vi "ROS_Read_Motors.vi"(7 "wl_in":T1={"topic port"=0, "Node"="", "topic"="", "type"="", "node port"=0, "error "={"status"=FALSE, "code"=0, "source"=""}, "Direction"=enum."Node", "Update (ms)"=1, "FIFO size"=1}, 8 "error in (no error)":errorcluster, 11 "wr_in":T1={"topic port"=0, "Node"="", "topic"="", "type"="", "node port"=0, "error "={"status"=FALSE, "code"=0, "source"=""}, "Direction"=enum."Node", "Update (ms)"=1, "FIFO size"=1}) -> (0 "error out":errorcluster, 1 "wr":sgl, 2 "wl":sgl, 3 "wr_out":T1={"topic port"=0, "Node"="", "topic"="", "type"="", "node port"=0, "error "={"status"=FALSE, "code"=0, "source"=""}, "Direction"=enum."Node", "Update (ms)"=1, "FIFO size"=1}, 5 "wl_out":T1={"topic port"=0, "Node"="", "topic"="", "type"="", "node port"=0, "error "={"status"=FALSE, "code"=0, "source"=""}, "Direction"=enum."Node", "Update (ms)"=1, "FIFO size"=1})   [LabVIEW 2017]
doc: "Read motors' left and right rotational velocity from ROS topics"
uses:
  <vilib>/Tufts CEEO ROS for LabVIEW Software/ROS/Code/SubVIs/_ROSControl.ctl
  <vilib>/Tufts CEEO ROS for LabVIEW Software/ROS/Code/SubVIs/_ROSDirection.ctl
  <vilib>/Tufts CEEO ROS for LabVIEW Software/ROS/MessageParsing/std_msgs/subs/parse_float32_scalar.vi
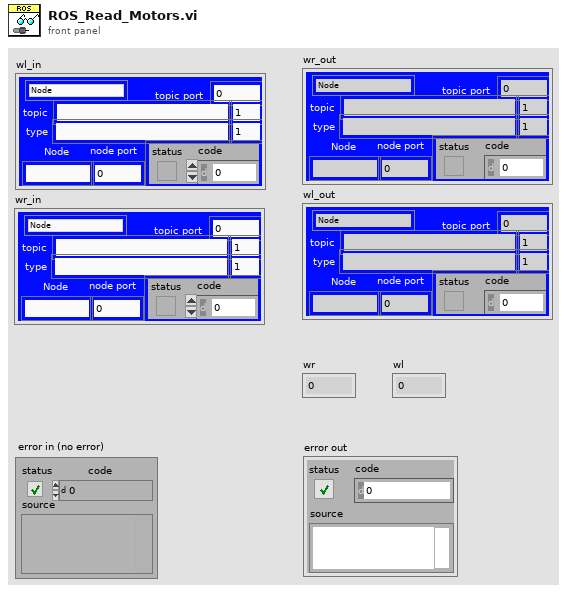
[diagram p1: front panel]
types:
  T1 = typedef "_ROSControl.ctl" = cluster{"topic port":u16, "Node":string, "topic":string, "type":string, "node port":u16, "error ":errorcluster, "Direction":T2, "Update (ms)":u16, "FIFO size":u16}
  T2 = typedef "_ROSDirection.ctl" = enum16{"Node", "Publisher", "Subscriber", "ServiceClient", "ServiceProvider"}
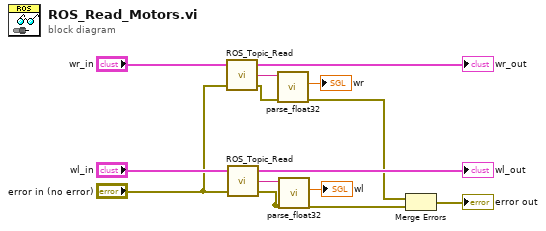
[diagram p0: block diagram]
diagram:
  n1 = call <vilib>:"ROS_Topic_Read.vi"("error in (no error)"="error in (no error)", "ROS in"="wr_in") -> ("error out"=w4:errorcluster, "Reply"=w8:string, "ROS out"=→"wr_out":T1)  [unwired: 1 in]
  n2 = call <vilib>:"ROS_Topic_Read.vi"("error in (no error)"="error in (no error)", "ROS in"="wl_in") -> ("error out"=w3:errorcluster, "Reply"=w7:string, "ROS out"=→"wl_out":T1)  [unwired: 1 in]
  n3 = call-poly <vilib>:"parse_float32.vi"("error in"=w4, "msg in"=w8) -> ("error out"=w2:errorcluster, "number"=→"wr":sgl)  [unwired: 3 in, 1 out]
  n4 = call-poly <vilib>:"parse_float32.vi"("error in"=w3, "msg in"=w7) -> ("number"=→"wl":sgl)  [unwired: 3 in, 2 out]
  n5 = Merge Errors(w2, w3) -> (→"error out":errorcluster)
